vi "ATZ.vi"(0 "System no.":i32=1 min=1 max=4 step=1, 2 "Affected axes":string[](array[string]), 3 "All axes?":bool, 4 "Low voltage":dbl[](array[numeric])=[nan, nan, nan, nan, nan, nan, nan] format="%.6f", 5 "error in":errorcluster, 12 "Stop refnum":refnum<vi>) -> (14 "ATZ successful?":bool[](array[boolean]), 19 "error out":errorcluster)   [LabVIEW 2020]
doc: "Performs an automatic zero-point calibration for the specified linear axes (see user manual for details), waits until this procedure has finished and returns whether ATZ was successful or not. Select NaN as Low voltage parameter if you want the controller to use the stored values it has. VI will also stop if Stop refnum or Local stop is TRUE. The home position is reset to default by ATZ. ATZ works independent of servo mode.\n\nC-413 : The result of the AutoZero procedure (new offset value) is present in RAM only. To save the result to EEPROM, where it becomes the power-on default, you must run WPA.vi. \n\nE-709: The result of the AutoZero procedure (new offset value) is present in RAM only. To save the result to EEPROM, where it becomes the power-on default, you must run WPA.vi. For stages with ID-chip the option \"Power Up Read ID-Chip\" must be disabled by default to make the AutoZero result available in the future. See E-709 user manual for details.\n\nE-712: The result of the AutoZero procedure (new offset value) is present in RAM only. To save the result to EEPROM, where it becomes the power-on default, you must run WPA.vi. For stages with ID-chip the option \"Power Up Read ID-Chip\" must be disabled by default to make the AutoZero result available in the future. See E-712 user manual for details.\n\nE-725, E-727: The result of the AutoZero procedure (new offset value) is present in RAM only. To save the result to EEPROM, where it becomes the power-on default, you must run WPA.vi. For stages with ID-chip the option \"Power Up Read ID-Chip\" must be disabled by default to make the AutoZero result available in the future. See controller user manual for details.\n\nE-753: The result of the AutoZero procedure (new offset value) is present in RAM only. To save the result to EEPROM, where it becomes the power-on default, you must run WPA.vi. For stages with ID-chip the option \"Power Up Read ID-Chip\" must be disabled by default to make the AutoZero result available in the future. See E-753 user manual for details.\n\nE-754: The result of the AutoZero procedure (new offset value) is present in RAM only. To save the result to EEPROM, where it becomes the power-on default, you must run WPA.vi. For stages with ID-chip the option \"Power Up Read ID-Chip\" must be disabled by default to make the AutoZero result available in the future. See E-754 user manual for details.\n\nE-761: Be aware that the result of the AutoZero procedure (new offset value) is automatically written to non-volatile memory (EPROM). For stages with ID-chip the option \"Read ID-Chip always\" must be disabled by default to make the AutoZero result (new offset value) available in the future. See E-761 user manual for details."
uses:
  Communication.llb/Global1.vi
panel:
  in  "Local stop":bool
  # "Performs automatic zero-point calibration  for specified linear axes, waits using \n#7 polling and indicates whether ATZ was successful or not. Select NaN as Low\nvoltage parameter if you want the controller to use the stored values it has. \nVI will also stop if Stop refnum or Local stop is TRUE."
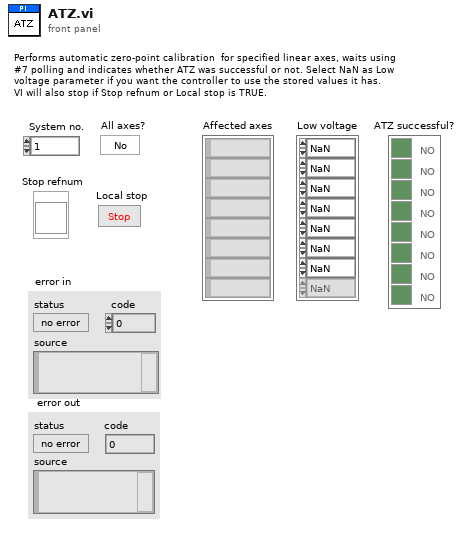
[diagram p1: front panel]
types:
  T1 = typedef "Syntax.ctl" = enum16{"GCS 1.0", "GCS 2.0", "GCS 3.0"}
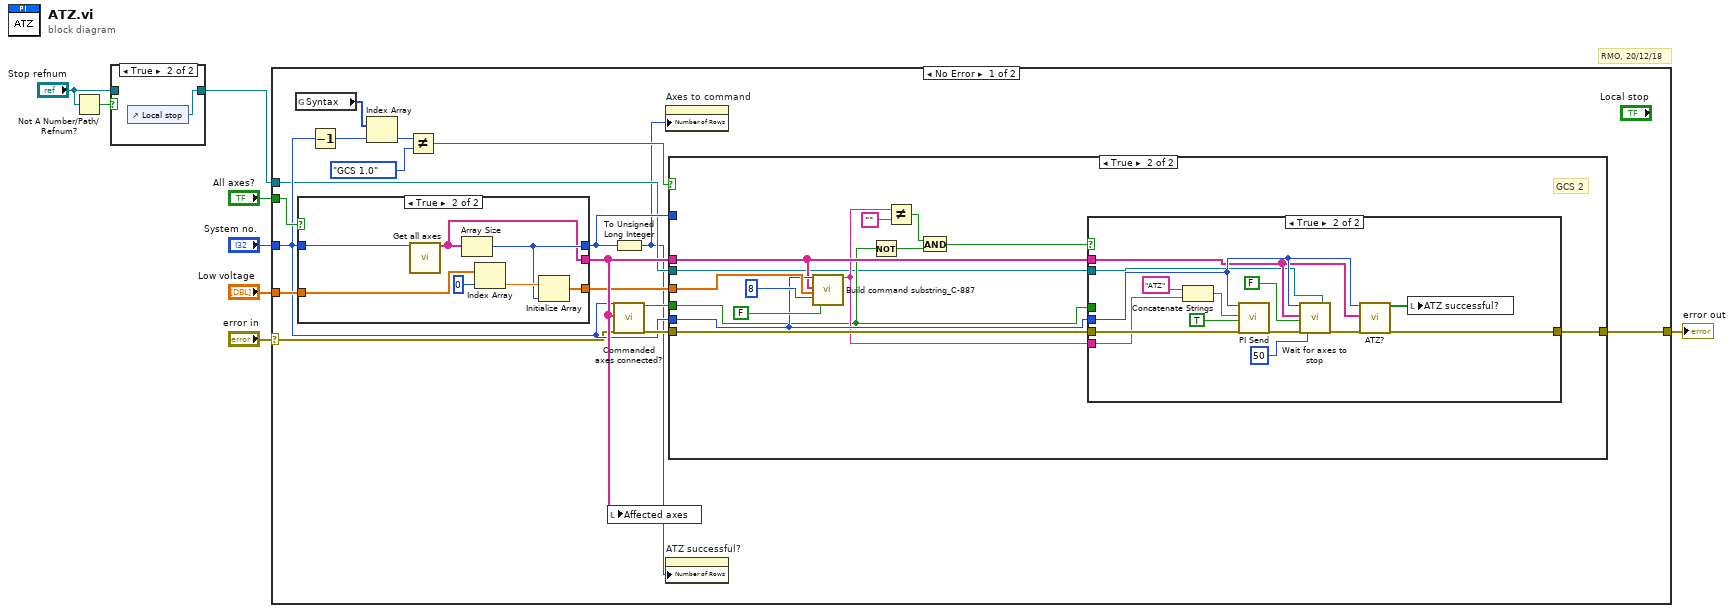
[diagram p0: block diagram]
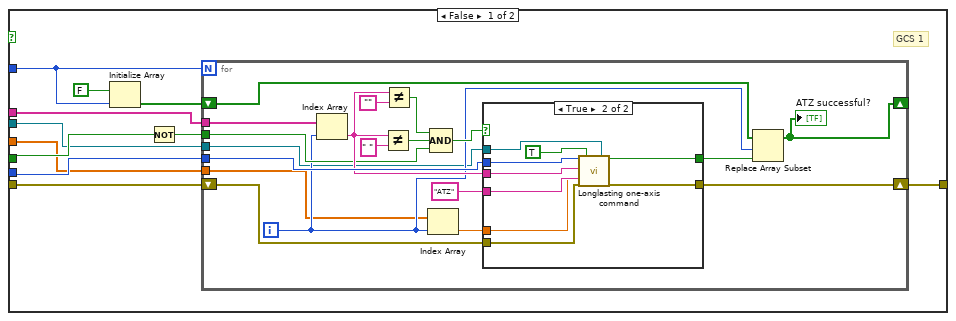
[diagram p3: hidden frame]
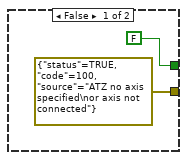
[diagram p4: hidden frame]
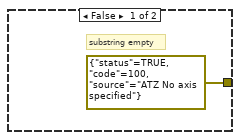
[diagram p6: hidden frame]
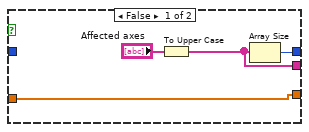
[diagram p7: hidden frame]
diagram:
  # "RMO, 20/12/18"
  n1 = Not A Number/Path/Refnum?(number/path/refnum="Stop refnum") -> (NaN/Path/Refnum?=w4:bool)
  n2 = case shown="True" w4 {
    tunnel: [w9 w10] -> w2
    tunnel: "Stop refnum" -> [w9 _]
    frame False {
    }
    frame True {
      n3 = control-ref of="Local stop"() -> (w10:refnum<vi>)
    }
  }
  n4 = case shown="No Error" "error in" {
    selector: "error in" -> [w11 w113]
    tunnel: "All axes?" -> [w27 _]
    tunnel: "System no." -> [w15 _]
    tunnel: [w26 w113] -> w6
    tunnel: "Low voltage" -> [w22 _]
    tunnel: w2 -> [w13 _]
    frame No Error {
      n5 = global read "Global1.vi" "Syntax"() -> (w16:T1[])
      n6 = case shown="True" w27 {
        tunnel: w15 -> [_ w107]
        tunnel: [w102 w106] -> w25
        tunnel: w22 -> [w104 w112]
        tunnel: [w103 w109] -> w21
        tunnel: [w104 w108] -> w20
        frame False {
          n7 = To Upper Case(1:"Affected axes") -> (0:w102:string[])
          n8 = Array Size(array=w102) -> (size(s)=w103:i32)
        }
        frame True {
          n9 = call "Get all axes.vi"("System no."=w107) -> ("Conn. Axes"=w106:string[])  [unwired: 18 out]
          n10 = Array Size(array=w106) -> (size(s)=w109:i32)
          n11 = Index Array(array=w112, index=0 ("Index")) -> (element=w110:dbl)
          n12 = Initialize Array(w110, w109) -> (w108:dbl[])
        }
      }
      n13 = Decrement(x=w15) -> (x-1=w17:i32)
      n14 = Index Array(array=w16, index=w17) -> (element=w18:T1)
      n15 = Not Equal?(x=w18, y=enum16{"GCS 1.0", "GCS 2.0"}."GCS 1.0") -> (x != y?=w14:bool)
      n16 = local write "Affected axes"(w25) -> ()
      n17 = To Unsigned Long Integer(number=w21) -> (unsigned 32bit integer=w12:u32)
      n18 = call "Commanded axes connected?.vi"("System no."=w15, "Commanded axes"=w25, "error in"=w11) -> ("Controller error"=w23:bool, "error out"=w24:errorcluster)  [unwired: 15 out]
      n19 = property on="Axes to command" class="Arr (strict)"("Number of Rows"=w12) -> ()  [unwired: 2 in, 2 out]
      n20 = property on="ATZ successful?" class="Arr (strict)"("Number of Rows"=w12) -> ()  [unwired: 2 in, 2 out]
      n21 = case shown="True" w14 {
        tunnel: [w36 w75] -> w26
        tunnel: w15 -> [w35 w74]
        tunnel: w25 -> [w34 w73]
        tunnel: w24 -> [w33 w76]
        tunnel: w23 -> [w32 w70]
        tunnel: w21 -> [w30 _]
        tunnel: w20 -> [w29 w79]
        tunnel: w13 -> [w28 w69]
        frame False {
          # "GCS 1"
          n22 = Initialize Array(FALSE, w30) -> (w37:bool[])
          n23 = Not(x=w32) -> (.not. x?=w31:bool)
          n24 = for {
            N: w30 -> [_]
            tunnel: w34 -> [w57]
            tunnel: w35 -> [w51]
            shift-right: [w49] -> w36
            shift-left: w33 -> [w48]
            shift-right: [w44] -> _
            shift-left: w37 -> [w45]
            tunnel: w31 -> [w43]
            tunnel: w29 -> [w41]
            tunnel: w28 -> [w39]
            i -> [w42]
            n25 = Index Array(array=w57, index=w42) -> (element=w50:string)
            n26 = Not Equal?(x=w50, y=" ") -> (x != y?=w53:bool)
            n27 = Not Equal?(x=w50, y="") -> (x != y?=w54:bool)
            n28 = Index Array(array=w41, index=w42) -> (element=w40:dbl)
            n29 = Compound Arithmetic op=AND(w54, w53, w43) -> (w52:bool)
            n30 = case shown="True" w52 {
              tunnel: w51 -> [_ w68]
              tunnel: w50 -> [_ w67]
              tunnel: [errorcluster {"status"=TRUE, "code"=100, "source"="ATZ no axis specified\nor axis not connected"} ("error out") w66] -> w49
              tunnel: w48 -> [_ w65]
              tunnel: "ATZ" -> [_ w64]
              tunnel: [FALSE w63] -> w46
              tunnel: w40 -> [_ w61]
              tunnel: w39 -> [_ w60]
              frame False {
              }
              frame True {
                n31 = call "Longlasting one-axis command.vi"("System no."=w68, "Axis to command"=w67, "Command"=w64, "Value"=w61, "error in"=w65, "Axis and value?"=TRUE, "Stop refnum"=w60) -> ("Answer"=w63:bool, "error out"=w66:errorcluster)  [unwired: 11 out]
              }
            }
            n32 = Replace Array Subset(array=w45, new element=w46, index=w42) -> (w44:bool[])
            "ATZ successful?" <- w44
          }
        }
        frame True {
          # "GCS 2"
          n33 = call "Build command substring_C-887.vi"("System no."=w74, "Affected axes"=w73, "Parameters"=w79, "No. of digits"=i16 8, "Parameter no. format \n(Decimal: FALSE)"=FALSE ("Parameter no. format \n(Decimal: FALSE)")) -> ("Command substring"=w71:string)  [unwired: 2 in, 12 out]
          n34 = Not(x=w70) -> (.not. x?=w80:bool)
          n35 = Not Equal?(x=w71, y="") -> (x != y?=w81:bool)
          n36 = And(x=w81, y=w80) -> (x .and. y?=w72:bool)
          n37 = case shown="True" w72 {
            tunnel: w76 -> [w84 w98]
            tunnel: [w83 w95] -> w75
            tunnel: w74 -> [_ w93]
            tunnel: w73 -> [_ w90]
            tunnel: w71 -> [_ w89]
            tunnel: w70 -> [w85 _]
            tunnel: w69 -> [_ w88]
            frame False {
              n38 = case shown="True" w85 {
                tunnel: [errorcluster {"status"=TRUE, "code"=100, "source"="ATZ No axis specified"} ("error out") w87] -> w83
                tunnel: w84 -> [_ w87]
                frame False {
                  # "substring empty"
                }
                frame True {
                  # "commanded axis not connected"
                }
              }
            }
            frame True {
              n39 = Concatenate Strings("ATZ", w89) -> (w100:string)
              n40 = call "PI Send.vi"("System no."=w93, "String to send"=w100, "Attach termination char.?"=TRUE, "error in"=w98) -> ("error out"=w97:errorcluster)  [unwired: 2 in, 13 out]
              n41 = call "Wait for axes to stop.vi"("System no."=w93, "Axes to wait for"=w90, "With status bit polling?"=FALSE, "error in"=w97, "Polling cycle time, ms"=u32 50, "Stop refnum"=w88) -> ("error out"=w96:errorcluster)  [unwired: 1 in, 12 out]
              n42 = call "ATZ?.vi"("System no."=w93, "Axes to query"=w90, "error in"=w96) -> ("ATZ successful?"=w94:bool[], "error out"=w95:errorcluster)  [unwired: 2 in, 13 out]
              n43 = local write "ATZ successful?"(w94) -> ()
            }
          }
        }
      }
    }
    frame Error {
    }
  }
  "error out" <- w6
